vi "System@ParameterSet__Parameter.vi"(1 "ParamterIn":string) -> (0 "ParamterOut":string)   [LabVIEW 2020]
panel:
  in  "Section":string(combo)
  in  "Value":string(combo)
  in  "ParameterName":string(combo)
  in  "Confirm":bool
  # "System@ParameterSet $Parameter,$Value(,$Section)"
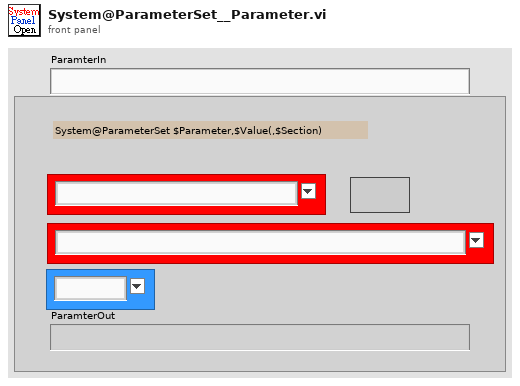
[diagram p1: front panel]
types:
  T1 = enum16{"Get", "Init", "Set", "Delete", "GetElement", "Inc", "Dec"}
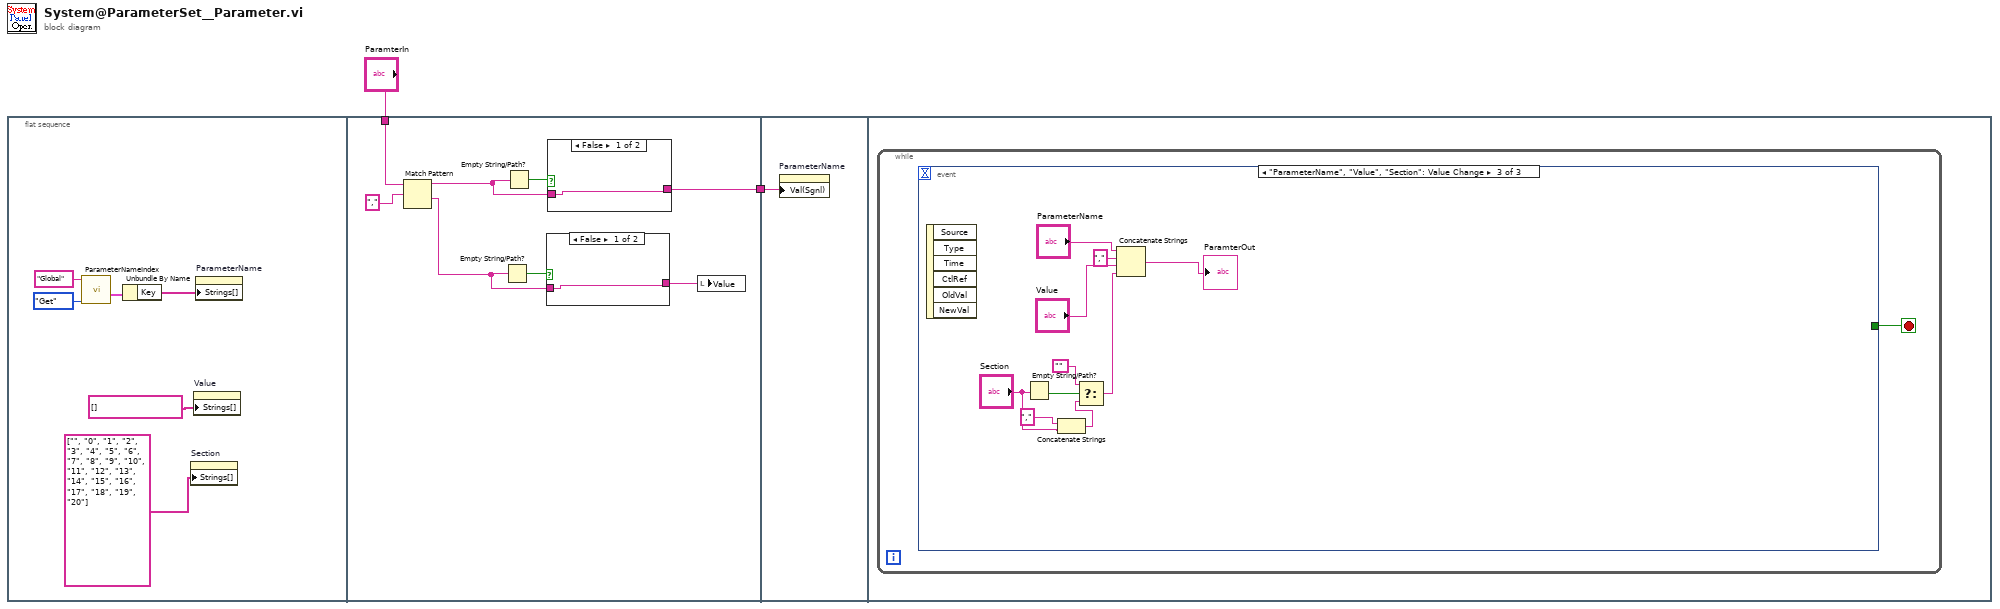
[diagram p0: block diagram]
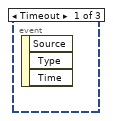
[diagram p4: hidden frame]
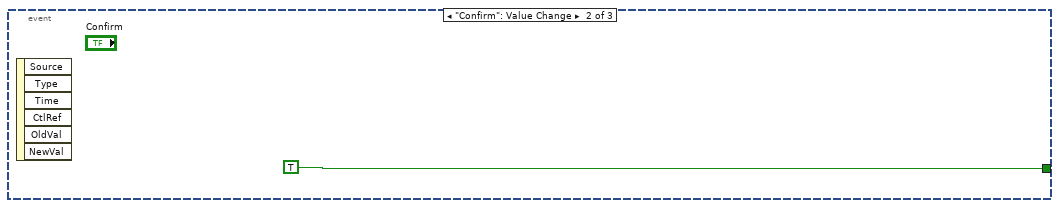
[diagram p5: hidden frame]
diagram:
  n1 = flat-sequence {
    tunnel: "ParamterIn" -> [w15]
    tunnel: [w10] -> w1
    tunnel: w1 -> [w21]
    frame #0 {
      n2 = call "ParameterNameIndex.vi"("OP"=T1."Get", "VariableSection"="Global") -> ("GlobalKeyValue"=w6:cluster{"Key":string[], "Value":string[]})  [unwired: 3 in, 6 out]
      n3 = Unbundle By Name(w6) -> ("Key"=w5:string[])
      n4 = property on="Section" class="CmbBox"("Strings[]"=string[] ["", "0", "1", "2", "3", "4", "5", "6", "7", "8", "9", "10", "11", "12", "13", "14", "15", "16", "17", "18", "19", "20"] ("Strings []")) -> ()  [unwired: 2 in, 2 out]
      n5 = property on="Value" class="CmbBox"("Strings[]"=string[] [] ("Strings []")) -> ()  [unwired: 2 in, 2 out]
      n6 = property on="ParameterName" class="CmbBox"("Strings[]"=w5) -> ()  [unwired: 2 in, 2 out]
    }
    frame #1 {
      n7 = Match Pattern(string=w15, regular expression=",") -> (before substring=w13:string, after substring=w11:string)  [unwired: 1 in, 2 out]
      n8 = Empty String/Path?(string/path=w11) -> (empty?=w12:bool)
      n9 = Empty String/Path?(string/path=w13) -> (empty?=w16:bool)
      n10 = case shown="False" w12 {
        tunnel: w11 -> [w17 w18]
        tunnel: [w17 w18] -> w9
        frame False {
        }
        frame True {
        }
      }
      n11 = case shown="False" w16 {
        tunnel: w13 -> [w19 w20]
        tunnel: [w19 w20] -> w10
        frame False {
        }
        frame True {
        }
      }
      n12 = local write "Value"(w9) -> ()
    }
    frame #2 {
      n13 = property on="ParameterName" class="CmbBox"("Val(Sgnl)"=w21) -> ()  [unwired: 2 in, 2 out]
    }
    frame #3 {
      n14 = while {
        stop <- w22 stop-if-true
        n15 = event shown="[2] \"ParameterName\", \"Value\", \"Section\": Value Change" {
          selector: _ -> [_ _ _]
          dyn-events: _ -> [_ _ _]
          timeout: _ -> [_ _ _]
          tunnel: [_ TRUE _] -> w22
          event Timeout {
            n16 = event-data() -> ()  [unwired: 1 in, 3 out]
          }
          event "Confirm": Value Change {
            n17 = event-data() -> ()  [unwired: 1 in, 6 out]
          }
          event "ParameterName", "Value", "Section": Value Change {
            n18 = event-data() -> ()  [unwired: 1 in, 6 out]
            n19 = Empty String/Path?(string/path="Section") -> (empty?=w29:bool)
            n20 = Concatenate Strings("," ("element"), "Section") -> (w27:string)
            n21 = Select(t="", s=w29, f=w27) -> (s? t:f=w24:string)
            n22 = Concatenate Strings("ParameterName", "," ("string"), "Value", w24) -> (→"ParamterOut":string)
          }
        }
      }
    }
  }
